vi "GeoData.vi"() -> ()   [LabVIEW 2017] (continued)
H1\n88058\t35013\tSan miguel\tNM\tDona Ana County\tH1\n88001\t35013\tLas cruces\tNM\tDona Ana County\tH1\n88011\t35013\tLas cruces\tNM\tDona Ana County\tH1\n88002\t35013\tWhite sands missile range\tNM\tDona Ana County\tH1\n88008\t35013\tSanta teresa\tNM\tDona Ana County\tH1\n88072\t35013\tVado\tNM\tDona Ana County\tH1\n88013\t35013\tLas cruces\tNM\tDona Ana County\tH1\n88046\t35013\tMesilla\tNM\tDona Ana County\tH1\n88052\t35013\tOrgan\tNM\tDona Ana County\tH1\n88033\t35013\tFairacres\tNM\tDona Ana County\tH1\n87936\t35013\tGarfield\tNM\tDona Ana County\tH1\n88032\t35013\tDona ana\tNM\tDona Ana County\tH1\n88048\t35013\tMesquite\tNM\tDona Ana County\tH1\n88003\t35013\tLas cruces\tNM\tDona Ana County\tH1\n87941\t35013\tSalem\tNM\tDona Ana County\tH1\n88012\t35013\tLas cruces\tNM\tDona Ana County\tH1\n88024\t35013\tBerino\tNM\tDona Ana County\tH1\n88210\t35015\tArtesia\tNM\tEddy County\tH1\n88253\t35015\tLake arthur\tNM\tEddy County\tH1\n88263\t35015\tMalaga\tNM\tEddy County\tH1\n88221\t35015\tCarlsbad\tNM\tEddy County\tH1\n88255\t35015\tLoco hills\tNM\tEddy County\tH1\n88250\t35015\tHope\tNM\tEddy County\tH1\n88268\t35015\tWhites city\tNM\tEddy County\tH1\n88220\t35015\tCarlsbad\tNM\tEddy County\tH1\n88256\t35015\tLoving\tNM\tEddy County\tH1\n88254\t35015\tLakewood\tNM\tEddy County\tH1\n88043\t35017\tHurley\tNM\tGrant County\tH1\n88023\t35017\tBayard\tNM\tGrant County\tH1\n88028\t35017\tCliff\tNM\tGrant County\tH1\n88026\t35017\tSanta clara\tNM\tGrant County\tH1\n88041\t35017\tHanover\tNM\tGrant County\tH1\n88049\t35017\tMimbres\tNM\tGrant County\tH1\n88062\t35017\tSilver city\tNM\tGrant County\tH1\n88055\t35017\tRedrock\tNM\tGrant County\tH1\n88065\t35017\tTyrone\tNM\tGrant County\tH1\n88061\t35017\tSilver city\tNM\tGrant County\tH1\n88025\t35017\tBuckhorn\tNM\tGrant County\tH1\n88034\t35017\tFaywood\tNM\tGrant County\tH1\n88051\t35017\tMule creek\tNM\tGrant County\tH1\n88036\t35017\tFort bayard\tNM\tGrant County\tH1\n88022\t35017\tArenas valley\tNM\tGrant County\tH1\n87821\t35017\tDatil\tNM\tGrant County\tH1\n88040\t35017\tHachita\tNM\tGrant County\tH1\n88053\t35017\tPinos altos\tNM\tGrant County\tH1\n88038\t35017\tGila\tNM\tGrant County\tH1\n88431\t35019\tNewkirk\tNM\tGuadalupe County\tH1\n88353\t35019\tVaughn\tNM\tGuadalupe County\tH1\n88417\t35019\tCuervo\tNM\tGuadalupe County\tH1\n87724\t35019\tLa loma\tNM\tGuadalupe County\tH1\n88435\t35019\tSanta rosa\tNM\tGuadalupe County\tH1\n87711\t35019\tAnton chico\tNM\tGuadalupe County\tH1\n87746\t35021\tSolano\tNM\tHarding County\tH1\n87733\t35021\tMosquero\tNM\tHarding County\tH1\n88415\t35021\tClayton\tNM\tHarding County\tH1\n88410\t35021\tAmistad\tNM\tHarding County\tH1\n88430\t35021\tNara visa\tNM\tHarding County\tH1\n88426\t35021\tLogan\tNM\tHarding County\tH1\n87730\t35021\tMills\tNM\tHarding County\tH1\n87743\t35021\tRoy\tNM\tHarding County\tH1\n88056\t35023\tRodeo\tNM\tHidalgo County\tH1\n88020\t35023\tAnimas\tNM\tHidalgo County\tH1\n88045\t35023\tLordsburg\tNM\tHidalgo County\tH1\n88267\t35025\tTatum\tNM\tLea County\tH1\n88260\t35025\tLovington\tNM\tLea County\tH1\n88213\t35025\tCaprock\tNM\tLea County\tH1\n88114\t35025\tCrossroads\tNM\tLea County\tH1\n88265\t35025\tMonument\tNM\tLea County\tH1\n88264\t35025\tMaljamar\tNM\tLea County\tH1\n88252\t35025\tJal\tNM\tLea County\tH1\n88241\t35025\tHobbs\tNM\tLea County\tH1\n88231\t35025\tEunice\tNM\tLea County\tH1\n88242\t35025\tHobbs\tNM\tLea County\tH1\n88240\t35025\tHobbs\tNM\tLea County\tH1\n88262\t35025\tMcdonald\tNM\tLea County\tH1\n88348\t35027\tSan patricio\tNM\tLincoln County\tH1\n88336\t35027\tHondo\tNM\tLincoln County\tH1\n88323\t35027\tFort stanton\tNM\tLincoln County\tH1\n88324\t35027\tGlencoe\tNM\tLincoln County\tH1\n88318\t35027\tCorona\tNM\tLincoln County\tH1\n88345\t35027\tRuidoso\tNM\tLincoln County\tH1\n88316\t35027\tCapitan\tNM\tLincoln County\tH1\n88355\t35027\tRuidoso\tNM\tLincoln County\tH1\n88301\t35027\tCarrizozo\tNM\tLincoln County\tH1\n88341\t35027\tNogal\tNM\tLincoln County\tH1\n88338\t35027\tLincoln\tNM\tLincoln County\tH1\n88346\t35027\tRuidoso downs\tNM\tLincoln County\tH1\n88312\t35027\tAlto\tNM\tLincoln County\tH1\n88351\t35027\tTinnie\tNM\tLincoln County\tH1\n88343\t35027\tPicacho\tNM\tLincoln County\tH1\n87547\t35028\tWhite rock\tNM\tLos Alamos County\tH1\n87544\t35028\tLos alamos\tNM\tLos Alamos County\tH1\n88030\t35029\tDeming\tNM\tLuna County\tH1\n88029\t35029\tColumbus\tNM\tLuna County\tH1\n88031\t35029\tDeming\tNM\tLuna County\tH1\n87020\t35031\tGrants\tNM\tMcKinley County\tH1\n87316\t35031\tFort wingate\tNM\tMcKinley County\tH1\n87328\t35031\tNavajo\tNM\tMcKinley County\tH1\n87313\t35031\tCrownpoint\tNM\tMcKinley County\tH1\n87319\t35031\tMentmore\tNM\tMcKinley County\tH1\n87323\t35031\tThoreau\tNM\tMcKinley County\tH1\n87321\t35031\tRamah\tNM\tMcKinley County\tH1\n87312\t35031\tContinental divide\tNM\tMcKinley County\tH1\n87311\t35031\tChurch rock\tNM\tMcKinley County\tH1\n87365\t35031\tSmith lake\tNM\tMcKinley County\tH1\n87322\t35031\tRehoboth\tNM\tMcKinley County\tH1\n87347\t35031\tJamestown\tNM\tMcKinley County\tH1\n87327\t35031\tZuni\tNM\tMcKinley County\tH1\n87045\t35031\tPrewitt\tNM\tMcKinley County\tH1\n87326\t35031\tVanderwagen\tNM\tMcKinley County\tH1\n87301\t35031\tGallup\tNM\tMcKinley County\tH1\n87305\t35031\tGallup\tNM\tMcKinley County\tH1\n87310\t35031\tBrimhall\tNM\tMcKinley County\tH1\n87302\t35031\tGallup\tNM\tMcKinley County\tH1\n87317\t35031\tGamerco\tNM\tMcKinley County\tH1\n87325\t35031\tTohatchi\tNM\tMcKinley County\tH1\n87320\t35031\tMexican springs\tNM\tMcKinley County\tH1\n87713\t35033\tChacon\tNM\tMora County\tH1\n87723\t35033\tHolman\tNM\tMora County\tH1\n87736\t35033\tRainsville\tNM\tMora County\tH1\n87715\t35033\tCleveland\tNM\tMora County\tH1\n87734\t35033\tOcate\tNM\tMora County\tH1\n87753\t35033\tWatrous\tNM\tMora County\tH1\n87752\t35033\tWagon mound\tNM\tMora County\tH1\n87732\t35033\tMora\tNM\tMora County\tH1\n87722\t35033\tGuadalupita\tNM\tMora County\tH1\n87735\t35033\tOjo feliz\tNM\tMora County\tH1\n87712\t35033\tBuena vista\tNM\tMora County\tH1\n87750\t35033\tValmora\tNM\tMora County\tH1\n88081\t35035\tChaparral\tNM\tOtero County\tH1\n88314\t35035\tBent\tNM\tOtero County\tH1\n88347\t35035\tSacramento\tNM\tOtero County\tH1\n88317\t35035\tCloudcroft\tNM\tOtero County\tH1\n88325\t35035\tHigh rolls mountain park\tNM\tOtero County\tH1\n88352\t35035\tTularosa\tNM\tOtero County\tH1\n88021\t35035\tAnthony\tNM\tOtero County\tH1\n88344\t35035\tPinon\tNM\tOtero County\tH1\n88340\t35035\tMescalero\tNM\tOtero County\tH1\n88350\t35035\tTimberon\tNM\tOtero County\tH1\n88310\t35035\tAlamogordo\tNM\tOtero County\tH1\n88311\t35035\tAlamogordo\tNM\tOtero County\tH1\n88349\t35035\tSunspot\tNM\tOtero County\tH1\n88342\t35035\tOrogrande\tNM\tOtero County\tH1\n88330\t35035\tHolloman air force base\tNM\tOtero County\tH1\n88337\t35035\tLa luz\tNM\tOtero County\tH1\n88339\t35035\tMayhill\tNM\tOtero County\tH1\n88354\t35035\tWeed\tNM\tOtero County\tH1\n88124\t35037\tMelrose\tNM\tQuay County\tH1\n88433\t35037\tQuay\tNM\tQuay County\tH1\n88120\t35037\tGrady\tNM\tQuay County\tH1\n88434\t35037\tSan jon\tNM\tQuay County\tH1\n88427\t35037\tMcalister\tNM\tQuay County\tH1\n88430\t35037\tNara visa\tNM\tQuay County\tH1\n88426\t35037\tLogan\tNM\tQuay County\tH1\n88411\t35037\tBard\tNM\tQuay County\tH1\n88121\t35037\tHouse\tNM\tQuay County\tH1\n88401\t35037\tTucumcari\tNM\tQuay County\tH1\n88112\t35037\tBroadview\tNM\tQuay County\tH1\n87528\t35039\tDulce\tNM\tRio Arriba County\tH1\n87531\t35039\tEmbudo\tNM\tRio Arriba County\tH1\n87029\t35039\tLindrith\tNM\tRio Arriba County\tH1\n87575\t35039\tTierra amarilla\tNM\tRio Arriba County\tH1\n87523\t35039\tCordova\tNM\tRio Arriba County\tH1\n87522\t35039\tChimayo\tNM\tRio Arriba County\tH1\n87510\t35039\tAbiquiu\tNM\tRio Arriba County\tH1\n87012\t35039\tCoyote\tNM\tRio Arriba County\tH1\n87532\t35039\tEspanola\tNM\tRio Arriba County\tH1\n87566\t35039\tOhkay owingeh\tNM\tRio Arriba County\tH1\n87530\t35039\tEl rito\tNM\tRio Arriba County\tH1\n87548\t35039\tMedanales\tNM\tRio Arriba County\tH1\n87554\t35039\tPetaca\tNM\tRio Arriba County\tH1\n87017\t35039\tGallina\tNM\tRio Arriba County\tH1\n87539\t35039\tLa madera\tNM\tRio Arriba County\tH1\n87520\t35039\tChama\tNM\tRio Arriba County\tH1\n87537\t35039\tHernandez\tNM\tRio Arriba County\tH1\n87551\t35039\tLos ojos\tNM\tRio Arriba County\tH1\n87582\t35039\tVelarde\tNM\tRio Arriba County\tH1\n87064\t35039\tYoungsville\tNM\tRio Arriba County\tH1\n87527\t35039\tDixon\tNM\tRio Arriba County\tH1\n87515\t35039\tCanjilon\tNM\tRio Arriba County\tH1\n87506\t35039\tSanta fe\tNM\tRio Arriba County\tH1\n87046\t35039\tRegina\tNM\tRio Arriba County\tH1\n87518\t35039\tCebolla\tNM\tRio Arriba County\tH1\n87412\t35039\tBlanco\tNM\tRio Arriba County\tH1\n87581\t35039\tVallecitos\tNM\tRio Arriba County\tH1\n87578\t35039\tTruchas\tNM\tRio Arriba County\tH1\n87516\t35039\tCanones\tNM\tRio Arriba County\tH1\n87511\t35039\tAlcalde\tNM\tRio Arriba County\tH1\n88115\t35041\tDora\tNM\tRoosevelt County\tH1\n88124\t35041\tMelrose\tNM\tRoosevelt County\tH1\n88134\t35041\tTaiban\tNM\tRoosevelt County\tH1\n88126\t35041\tPep\tNM\tRoosevelt County\tH1\n88123\t35041\tLingo\tNM\tRoosevelt County\tH1\n88101\t35041\tClovis\tNM\tRoosevelt County\tH1\n88130\t35041\tPortales\tNM\tRoosevelt County\tH1\n88114\t35041\tCrossroads\tNM\tRoosevelt County\tH1\n88113\t35041\tCausey\tNM\tRoosevelt County\tH1\n88125\t35041\tMilnesand\tNM\tRoosevelt County\tH1\n88116\t35041\tElida\tNM\tRoosevelt County\tH1\n88132\t35041\tRogers\tNM\tRoosevelt County\tH1\n88122\t35041\tKenna\tNM\tRoosevelt County\tH1\n88135\t35041\tTexico\tNM\tRoosevelt County\tH1\n88118\t35041\tFloyd\tNM\tRoosevelt County\tH1\n87041\t35043\tPena blanca\tNM\tSandoval County\tH1\n87072\t35043\tCochiti pueblo\tNM\tSandoval County\tH1\n87047\t35043\tSandia park\tNM\tSandoval County\tH1\n87048\t35043\tCorrales\tNM\tSandoval County\tH1\n87544\t35043\tLos alamos\tNM\tSandoval County\tH1\n87025\t35043\tJemez springs\tNM\tSandoval County\tH1\n87053\t35043\tSan ysidro\tNM\tSandoval County\tH1\n87122\t35043\tAlbuquerque\tNM\tSandoval County\tH1\n87174\t35043\tRio rancho\tNM\tSandoval County\tH1\n87124\t35043\tRio rancho\tNM\tSandoval County\tH1\n87027\t35043\tLa jara\tNM\tSandoval County\tH1\n87044\t35043\tPonderosa\tNM\tSandoval County\tH1\n87004\t35043\tBernalillo\tNM\tSandoval County\tH1\n87024\t35043\tJemez pueblo\tNM\tSandoval County\tH1\n87001\t35043\tAlgodones\tNM\tSandoval County\tH1\n87083\t35043\tCochiti lake\tNM\tSandoval County\tH1\n87043\t35043\tPlacitas\tNM\tSandoval County\tH1\n87052\t35043\tSanto domingo pueblo\tNM\tSandoval County\tH1\n87018\t35043\tCounselor\tNM\tSandoval County\tH1\n87046\t35043\tRegina\tNM\tSandoval County\tH1\n87144\t35043\tRio rancho\tNM\tSandoval County\tH1\n87013\t35043\tCuba\tNM\tSandoval County\tH1\n87402\t35045\tFarmington\tNM\tSan Juan County\tH1\n87499\t35045\tFarmington\tNM\tSan Juan County\tH1\n87418\t35045\tLa plata\tNM\tSan Juan County\tH1\n87455\t35045\tNewcomb\tNM\tSan Juan County\tH1\n87421\t35045\tWaterflow\tNM\tSan Juan County\tH1\n87419\t35045\tNavajo dam\tNM\tSan Juan County\tH1\n87461\t35045\tSanostee\tNM\tSan Juan County\tH1\n87413\t35045\tBloomfield\tNM\tSan Juan County\tH1\n87420\t35045\tShiprock\tNM\tSan Juan County\tH1\n87416\t35045\tFruitland\tNM\tSan Juan County\tH1\n87417\t35045\tKirtland\tNM\tSan Juan County\tH1\n87364\t35045\tSheep springs\tNM\tSan Juan County\tH1\n87037\t35045\tNageezi\tNM\tSan Juan County\tH1\n87412\t35045\tBlanco\tNM\tSan Juan County\tH1\n87401\t35045\tFarmington\tNM\tSan Juan County\tH1\n87410\t35045\tAztec\tNM\tSan Juan County\tH1\n87415\t35045\tFlora vista\tNM\tSan Juan County\tH1\n87565\t35047\tSan jose\tNM\tSan Miguel County\tH1\n87746\t35047\tSolano\tNM\tSan Miguel County\tH1\n87583\t35047\tVillanueva\tNM\tSan Miguel County\tH1\n88421\t35047\tGarita\tNM\tSan Miguel County\tH1\n87569\t35047\tSerafina\tNM\tSan Miguel County\tH1\n87538\t35047\tIlfeld\tNM\tSan Miguel County\tH1\n87560\t35047\tRibera\tNM\tSan Miguel County\tH1\n87573\t35047\tTererro\tNM\tSan Miguel County\tH1\n87701\t35047\tLas vegas\tNM\tSan Miguel County\tH1\n87552\t35047\tPecos\tNM\tSan Miguel County\tH1\n88439\t35047\tTrementina\tNM\tSan Miguel County\tH1\n87562\t35047\tRowe\tNM\tSan Miguel County\tH1\n87731\t35047\tMontezuma\tNM\tSan Miguel County\tH1\n88416\t35047\tConchas dam\tNM\tSan Miguel County\tH1\n87711\t35047\tAnton chico\tNM\tSan Miguel County\tH1\n87535\t35047\tGlorieta\tNM\tSan Miguel County\tH1\n87745\t35047\tSapello\tNM\tSan Miguel County\tH1\n87742\t35047\tRociada\tNM\tSan Miguel County\tH1\n87035\t35049\tMoriarty\tNM\tSanta Fe County\tH1\n87502\t35049\tSanta fe\tNM\tSanta Fe County\tH1\n87015\t35049\tEdgewood\tNM\tSanta Fe County\tH1\n87047\t35049\tSandia park\tNM\tSanta Fe County\tH1\n87504\t35049\tSanta fe\tNM\tSanta Fe County\tH1\n87522\t35049\tChimayo\tNM\tSanta Fe County\tH1\n87567\t35049\tSanta cruz\tNM\tSanta Fe County\tH1\n87505\t35049\tSanta fe\tNM\tSanta Fe County\tH1\n87532\t35049\tEspanola\tNM\tSanta Fe County\tH1\n87592\t35049\tSanta fe\tNM\tSanta Fe County\tH1\n87501\t35049\tSanta fe\tNM\tSanta Fe County\tH1\n87540\t35049\tLamy\tNM\tSanta Fe County\tH1\n87010\t35049\tCerrillos\tNM\tSanta Fe County\tH1\n87508\t35049\tSanta fe\tNM\tSanta Fe County\tH1\n87552\t35049\tPecos\tNM\tSanta Fe County\tH1\n87506\t35049\tSanta fe\tNM\tSanta Fe County\tH1\n87507\t35049\tSanta fe\tNM\tSanta Fe County\tH1\n87594\t35049\tSanta fe\tNM\tSanta Fe County\tH1\n87056\t35049\tStanley\tNM\tSanta Fe County\tH1\n87574\t35049\tTesuque\tNM\tSanta Fe County\tH1\n87535\t35049\tGlorieta\tNM\tSanta Fe County\tH1\n87901\t35051\tTruth or consequences\tNM\tSierra County\tH1\n87942\t35051\tWilliamsburg\tNM\tSierra County\tH1\n87654\t35051\tSpaceport city\tNM\tSierra County\tH1\n87930\t35051\tArrey\tNM\tSierra County\tH1\n87933\t35051\tDerry\tNM\tSierra County\tH1\n87943\t35051\tWinston\tNM\tSierra County\tH1\n87931\t35051\tCaballo\tNM\tSierra County\tH1\n87935\t35051\tElephant butte\tNM\tSierra County\tH1\n88042\t35051\tHillsboro\tNM\tSierra County\tH1\n87939\t35051\tMonticello\tNM\tSierra County\tH1\n87823\t35053\tLemitar\tNM\tSocorro County\tH1\n87825\t35053\tMagdalena\tNM\tSocorro County\tH1\n87801\t35053\tSocorro\tNM\tSocorro County\tH1\n87028\t35053\tLa joya\tNM\tSocorro County\tH1\n87011\t35053\tClaunch\tNM\tSocorro County\tH1\n87062\t35053\tVeguita\tNM\tSocorro County\tH1\n87006\t35053\tBosque\tNM\tSocorro County\tH1\n87828\t35053\tPolvadera\tNM\tSocorro County\tH1\n87831\t35053\tSan acacia\tNM\tSocorro County\tH1\n87832\t35053\tSan antonio\tNM\tSocorro County\tH1\n87514\t35055\tArroyo seco\tNM\tTaos County\tH1\n87524\t35055\tCostilla\tNM\tTaos County\tH1\n87577\t35055\tTres piedras\tNM\tTaos County\tH1\n87576\t35055\tTrampas\tNM\tTaos County\tH1\n87579\t35055\tVadito\tNM\tTaos County\tH1\n87580\t35055\tValdez\tNM\tTaos County\tH1\n87525\t35055\tTaos ski valley\tNM\tTaos County\tH1\n87571\t35055\tTaos\tNM\tTaos County\tH1\n87519\t35055\tCerro\tNM\tTaos County\tH1\n87543\t35055\tLlano\tNM\tTaos County\tH1\n87512\t35055\tAmalia\tNM\tTaos County\tH1\n87553\t35055\tPenasco\tNM\tTaos County\tH1\n87558\t35055\tRed river\tNM\tTaos County\tH1\n87549\t35055\tOjo caliente\tNM\tTaos County\tH1\n87557\t35055\tRanchos de taos\tNM\tTaos County\tH1\n87529\t35055\tEl prado\tNM\tTaos County\tH1\n87521\t35055\tChamisal\tNM\tTaos County\tH1\n87513\t35055\tArroyo hondo\tNM\tTaos County\tH1\n87517\t35055\tCarson\tNM\tTaos County\tH1\n87564\t35055\tSan cristobal\tNM\tTaos County\tH1\n87556\t35055\tQuesta\tNM\tTaos County\tH1\n87035\t35057\tMoriarty\tNM\tTorrance County\tH1\n87015\t35057\tEdgewood\tNM\tTorrance County\tH1\n87061\t35057\tTorreon\tNM\tTorrance County\tH1\n87070\t35057\tClines corners\tNM\tTorrance County\tH1\n88321\t35057\tEncino\tNM\tTorrance County\tH1\n87009\t35057\tCedarvale\tNM\tTorrance County\tH1\n87016\t35057\tEstancia\tNM\tTorrance County\tH1\n87036\t35057\tMountainair\tNM\tTorrance County\tH1\n87063\t35057\tWillard\tNM\tTorrance County\tH1\n87032\t35057\tMcintosh\tNM\tTorrance County\tH1\n88414\t35059\tCapulin\tNM\tUnion County\tH1\n88415\t35059\tClayton\tNM\tUnion County\tH1\n88410\t35059\tAmistad\tNM\tUnion County\tH1\n88422\t35059\tGladstone\tNM\tUnion County\tH1\n88419\t35059\tFolsom\tNM\tUnion County\tH1\n88418\t35059\tDes moines\tNM\tUnion County\tH1\n88430\t35059\tNara visa\tNM\tUnion County\tH1\n88436\t35059\tSedan\tNM\tUnion County\tH1\n88424\t35059\tGrenville\tNM\tUnion County\tH1\n87031\t35061\tLos lunas\tNM\tValencia County\tH1\n87068\t35061\tBosque farms\tNM\tValencia County\tH1\n87060\t35061\tTome\tNM\tValencia County\tH1\n87042\t35061\tPeralta\tNM\tValencia County\tH1\n87062\t35061\tVeguita\tNM\tValencia County\tH1\n87006\t35061\tBosque\tNM\tValencia County\tH1\n87002\t35061\tBelen\tNM\tValencia County\tH1\n87026\t35061\tLaguna\tNM\tValencia County\tH1\n87023\t35061\tJarales\tNM\tValencia County\tH1\n12087\t36001\tHannacroix\tNY\tAlbany County\tH1\n12189\t36001\tWatervliet\tNY\tAlbany County\tH1\n12204\t36001\tAlbany\tNY\tAlbany County\tH1\n12207\t36001\tAlbany\tNY\tAlbany County\tH1\n12226\t36001\tAlbany\tNY\tAlbany County\tH1\n12234\t36001\tAlbany\tNY\tAlbany County\tH1\n12232\t36001\tAlbany\tNY\tAlbany County\tH1\n12055\t36001\tDormansville\tNY\tAlbany County\tH1\n12469\t36001\tPreston hollow\tNY\tAlbany County\tH1\n12047\t36001\tCohoes\tNY\tAlbany County\tH1\n12157\t36001\tSchoharie\tNY\tAlbany County\tH1\n12183\t36001\tTroy\tNY\tAlbany County\tH1\n12007\t36001\tAlcove\tNY\tAlbany County\tH1\n12041\t36001\tClarksville\tNY\tAlbany County\tH1\n12255\t36001\tAlbany\tNY\tAlbany County\tH1\n12460\t36001\tOak hill\tNY\tAlbany County\tH1\n12023\t36001\tBerne\tNY\tAlbany County\tH1\n12053\t36001\tDelanson\tNY\tAlbany County\tH1\n12161\t36001\tSouth bethlehem\tNY\tAlbany County\tH1\n12122\t36001\tMiddleburgh\tNY\tAlbany County\tH1\n12206\t36001\tAlbany\tNY\tAlbany County\tH1\n12306\t36001\tSchenectady\tNY\tAlbany County\tH1\n12257\t36001\tAlbany\tNY\tAlbany County\tH1\n12107\t36001\tKnox\tNY\tAlbany County\tH1\n12245\t36001\tAlbany\tNY\tAlbany County\tH1\n12083\t36001\tGreenville\tNY\tAlbany County\tH1\n12158\t36001\tSelkirk\tNY\tAlbany County\tH1\n12205\t36001\tAlbany\tNY\tAlbany County\tH1\n12309\t36001\tSchenectady\tNY\tAlbany County\tH1\n12247\t36001\tAlbany\tNY\tAlbany County\tH1\n12223\t36001\tAlbany\tNY\tAlbany County\tH1\n12222\t36001\tAlbany\tNY\tAlbany County\tH1\n12260\t36001\tAlbany\tNY\tAlbany County\tH1\n12235\t36001\tAlbany\tNY\tAlbany County\tH1\n12249\t36001\tAlbany\tNY\tAlbany County\tH1\n12110\t36001\tLatham\tNY\tAlbany County\tH1\n12159\t36001\tSlingerlands\tNY\tAlbany County\tH1\n12202\t36001\tAlbany\tNY\tAlbany County\tH1\n12193\t36001\tWesterlo\tNY\tAlbany County\tH1\n12067\t36001\tFeura bush\tNY\tAlbany County\tH1\n12077\t36001\tGlenmont\tNY\tAlbany County\tH1\n12084\t36001\tGuilderland\tNY\tAlbany County\tH1\n12059\t36001\tEast berne\tNY\tAlbany County\tH1\n12147\t36001\tRensselaerville\tNY\tAlbany County\tH1\n12143\t36001\tRavena\tNY\tAlbany County\tH1\n12186\t36001\tVoorheesville\tNY\tAlbany County\tH1\n12209\t36001\tAlbany\tNY\tAlbany County\tH1\n12303\t36001\tSchenectady\tNY\tAlbany County\tH1\n12304\t36001\tSchenectady\tNY\tAlbany County\tH1\n12045\t36001\tCoeymans\tNY\tAlbany County\tH1\n12120\t36001\tMedusa\tNY\tAlbany County\tH1\n12085\t36001\tGuilderland center\tNY\tAlbany County\tH1\n12240\t36001\tAlbany\tNY\tAlbany County\tH1\n12248\t36001\tAlbany\tNY\tAlbany County\tH1\n12128\t36001\tNewtonville\tNY\tAlbany County\tH1\n12224\t36001\tAlbany\tNY\tAlbany County\tH1\n12009\t36001\tAltamont\tNY\tAlbany County\tH1\n12208\t36001\tAlbany\tNY\tAlbany County\tH1\n12212\t36001\tAlbany\tNY\tAlbany County\tH1\n12201\t36001\tAlbany\tNY\tAlbany County\tH1\n12236\t36001\tAlbany\tNY\tAlbany County\tH1\n12054\t36001\tDelmar\tNY\tAlbany County\tH1\n12065\t36001\tClifton park\tNY\tAlbany County\tH1\n12203\t36001\tAlbany\tNY\tAlbany County\tH1\n12211\t36001\tAlbany\tNY\tAlbany County\tH1\n12210\t36001\tAlbany\tNY\tAlbany County\tH1\n12046\t36001\tCoeymans hollow\tNY\tAlbany County\tH1\n12220\t36001\tAlbany\tNY\tAlbany County\tH1\n12246\t36001\tAlbany\tNY\tAlbany County\tH1\n12237\t36001\tAlbany\tNY\tAlbany County\tH1\n12288\t36001\tAlbany\tNY\tAlbany County\tH1\n12227\t36001\tAlbany\tNY\tAlbany County\tH1\n14717\t36003\tCaneadea\tNY\tAllegany County\tH1\n14802\t36003\tAlfred\tNY\tAllegany County\tH1\n14060\t36003\tFarmersville station\tNY\tAllegany County\tH1\n14721\t36003\tCeres\tNY\tAllegany County\tH1\n14745\t36003\tHume\tNY\tAllegany County\tH1\n14065\t36003\tFreedom\tNY\tAllegany County\tH1\n14822\t36003\tCanaseraga\tNY\tAllegany County\tH1\n14836\t36003\tDalton\tNY\tAllegany County\tH1\n14843\t36003\tHornell\tNY\tAllegany County\tH1\n14897\t36003\tWhitesville\tNY\tAllegany County\tH1\n14029\t36003\tCenterville\tNY\tAllegany County\tH1\n14774\t36003\tRichburg\tNY\tAllegany County\tH1\n14754\t36003\tLittle genesee\tNY\tAllegany County\tH1\n14709\t36003\tAngelica\tNY\tAllegany County\tH1\n14884\t36003\tSwain\tNY\tAllegany County\tH1\n14714\t36003\tBlack creek\tNY\tAllegany County\tH1\n14895\t36003\tWellsville\tNY\tAllegany County\tH1\n14806\t36003\tAndover\tNY\tAllegany County\tH1\n14786\t36003\tWest clarksville\tNY\tAllegany County\tH1\n14437\t36003\tDansville\tNY\tAllegany County\tH1\n14803\t36003\tAlfred station\tNY\tAllegany County\tH1\n14715\t36003\tBolivar\tNY\tAllegany County\tH1\n14708\t36003\tAlma\tNY\tAllegany County\tH1\n14024\t36003\tBliss\tNY\tAllegany County\tH1\n14727\t36003\tCuba\tNY\tAllegany County\tH1\n14770\t36003\tPortville\tNY\tAllegany County\tH1\n14807\t36003\tArkport\tNY\tAllegany County\tH1\n14739\t36003\tFriendship\tNY\tAllegany County\tH1\n14846\t36003\tHunt\tNY\tAllegany County\tH1\n14744\t36003\tHoughton\tNY\tAllegany County\tH1\n14707\t36003\tAllentown\tNY\tAllegany County\tH1\n14737\t36003\tFranklinville\tNY\tAllegany County\tH1\n14813\t36003\tBelmont\tNY\tAllegany County\tH1\n14735\t36003\tFillmore\tNY\tAllegany County\tH1\n14880\t36003\tScio\tNY\tAllegany County\tH1\n14777\t36003\tRushford\tNY\tAllegany County\tH1\n14804\t36003\tAlmond\tNY\tAllegany County\tH1\n14711\t36003\tBelfast\tNY\tAllegany County\tH1\n14536\t36003\tPortageville\tNY\tAllegany County\tH1\n10459\t36005\tBronx\tNY\tBronx County\tH6\n10457\t36005\tBronx\tNY\tBronx County\tH6\n10455\t36005\tBronx\tNY\tBronx County\tH6\n10465\t36005\tBronx\tNY\tBronx County\tH6\n10468\t36005\tBronx\tNY\tBronx County\tH6\n10466\t36005\tBronx\tNY\tBronx County\tH6\n10473\t36005\tBronx\tNY\tBronx County\tH6\n10550\t36005\tMount vernon\tNY\tBronx County\tH6\n10458\t36005\tBronx\tNY\tBronx County\tH6\n10463\t36005\tBronx\tNY\tBronx County\tH6\n10464\t36005\tBronx\tNY\tBronx County\tH6\n10469\t36005\tBronx\tNY\tBronx County\tH6\n10453\t36005\tBronx\tNY\tBronx County\tH6\n10460\t36005\tBronx\tNY\tBronx County\tH6\n10461\t36005\tBronx\tNY\tBronx County\tH6\n10462\t36005\tBronx\tNY\tBronx County\tH6\n10471\t36005\tBronx\tNY\tBronx County\tH6\n10454\t36005\tBronx\tNY\tBronx County\tH6\n10456\t36005\tBronx\tNY\tBronx County\tH6\n10467\t36005\tBronx\tNY\tBronx County\tH6\n10470\t36005\tBronx\tNY\tBronx County\tH6\n10475\t36005\tBronx\tNY\tBronx County\tH6\n10472\t36005\tBronx\tNY\tBronx County\tH6\n10474\t36005\tBronx\tNY\tBronx County\tH6\n10705\t36005\tYonkers\tNY\tBronx County\tH6\n10452\t36005\tBronx\tNY\tBronx County\tH6\n10451\t36005\tBronx\tNY\tBronx County\tH6\n10803\t36005\tPelham\tNY\tBronx County\tH6\n13746\t36007\tChenango forks\tNY\tBroome County\tH1\n13730\t36007\tAfton\tNY\tBroome County\tH1\n13787\t36007\tHarpursville\tNY\tBroome County\tH1\n13850\t36007\tVestal\tNY\tBroome County\tH1\n13901\t36007\tBinghamton\tNY\tBroome County\tH1\n13835\t36007\tRichford\tNY\tBroome County\tH1\n13813\t36007\tNineveh\tNY\tBroome County\tH1\n13732\t36007\tApalachin\tNY\tBroome County\tH1\n13778\t36007\tGreene\tNY\tBroome County\tH1\n13761\t36007\tEndicott\tNY\tBroome County\tH1\n13797\t36007\tLisle\tNY\tBroome County\tH1\n13803\t36007\tMarathon\tNY\tBroome County\tH1\n13777\t36007\tGlen aubrey\tNY\tBroome County\tH1\n13737\t36007\tBible school park\tNY\tBroome County\tH1\n13790\t36007\tJohnson city\tNY\tBroome County\tH1\n13902\t36007\tBinghamton\tNY\tBroome County\tH1\n13762\t36007\tEndwell\tNY\tBroome County\tH1\n13754\t36007\tDeposit\tNY\tBroome County\tH1\n13736\t36007\tBerkshire\tNY\tBroome County\tH1\n13811\t36007\tNewark valley\tNY\tBroome County\tH1\n13745\t36007\tChenango bridge\tNY\tBroome County\tH1\n13794\t36007\tKillawog\tNY\tBroome County\tH1\n13851\t36007\tVestal\tNY\tBroome County\tH1\n13833\t36007\tPort crane\tNY\tBroome County\tH1\n13904\t36007\tBinghamton\tNY\tBroome County\tH1\n13795\t36007\tKirkwood\tNY\tBroome County\tH1\n13748\t36007\tConklin\tNY\tBroome County\tH1\n13760\t36007\tEndicott\tNY\tBroome County\tH1\n13802\t36007\tMaine\tNY\tBroome County\tH1\n13862\t36007\tWhitney point\tNY\tBroome County\tH1\n13826\t36007\tOuaquaga\tNY\tBroome County\tH1\n13783\t36007\tHancock\tNY\tBroome County\tH1\n13744\t36007\tCastle creek\tNY\tBroome County\tH1\n13903\t36007\tBinghamton\tNY\tBroome County\tH1\n13905\t36007\tBinghamton\tNY\tBroome County\tH1\n13865\t36007\tWindsor\tNY\tBroome County\tH1\n13863\t36007\tWillet\tNY\tBroome County\tH1\n13848\t36007\tTunnel\tNY\tBroome County\tH1\n13749\t36007\tCorbettsville\tNY\tBroome County\tH1\n14738\t36009\tFrewsburg\tNY\tCattaraugus County\tH1\n14755\t36009\tLittle valley\tNY\tCattaraugus County\tH1\n14134\t36009\tSardinia\tNY\tCattaraugus County\tH1\n14030\t36009\tChaffee\tNY\tCattaraugus County\tH1\n14060\t36009\tFarmersville station\tNY\tCattaraugus County\tH1\n14041\t36009\tDayton\tNY\tCattaraugus County\tH1\n14751\t36009\tLeon\tNY\tCattaraugus County\tH1\n14065\t36009\tFreedom\tNY\tCattaraugus County\tH1\n14729\t36009\tEast otto\tNY\tCattaraugus County\tH1\n14753\t36009\tLimestone\tNY\tCattaraugus County\tH1\n14766\t36009\tOtto\tNY\tCattaraugus County\tH1\n14101\t36009\tMachias\tNY\tCattaraugus County\tH1\n14747\t36009\tKennedy\tNY\tCattaraugus County\tH1\n14779\t36009\tSalamanca\tNY\tCattaraugus County\tH1\n14129\t36009\tPerrysburg\tNY\tCattaraugus County\tH1\n14778\t36009\tSaint bonaventure\tNY\tCattaraugus County\tH1\n14042\t36009\tDelevan\tNY\tCattaraugus County\tH1\n14719\t36009\tCattaraugus\tNY\tCattaraugus County\tH1\n14760\t36009\tOlean\tNY\tCattaraugus County\tH1\n14081\t36009\tIrving\tNY\tCattaraugus County\tH1\n14171\t36009\tWest valley\tNY\tCattaraugus County\tH1\n14706\t36009\tAllegany\tNY\tCattaraugus County\tH1\n14070\t36009\tGowanda\tNY\tCattaraugus County\tH1\n14062\t36009\tForestville\tNY\tCattaraugus County\tH1\n14138\t36009\tSouth dayton\tNY\tCattaraugus County\tH1\n14748\t36009\tKill buck\tNY\tCattaraugus County\tH1\n14783\t36009\tSteamburg\tNY\tCattaraugus County\tH1\n14730\t36009\tEast randolph\tNY\tCattaraugus County\tH1\n14727\t36009\tCuba\tNY\tCattaraugus County\tH1\n14770\t36009\tPortville\tNY\tCattaraugus County\tH1\n14788\t36009\tWestons mills\tNY\tCattaraugus County\tH1\n14009\t36009\tArcade\tNY\tCattaraugus County\tH1\n14737\t36009\tFranklinville\tNY\tCattaraugus County\tH1\n14726\t36009\tConewango valley\tNY\tCattaraugus County\tH1\n14743\t36009\tHinsdale\tNY\tCattaraugus County\tH1\n14741\t36009\tGreat valley\tNY\tCattaraugus County\tH1\n14173\t36009\tYorkshire\tNY\tCattaraugus County\tH1\n14141\t36009\tSpringville\tNY\tCattaraugus County\tH1\n14731\t36009\tEllicottville\tNY\tCattaraugus County\tH1\n14772\t36009\tRandolph\tNY\tCattaraugus County\tH1\n14168\t36009\tVersailles\tNY\tCattaraugus County\tH1\n13074\t36011\tHannibal\tNY\tCayuga County\tH1\n13092\t36011\tLocke\tNY\tCayuga County\tH1\n13111\t36011\tMartville\tNY\tCayuga County\tH1\n13143\t36011\tRed creek\tNY\tCayuga County\tH1\n13166\t36011\tWeedsport\tNY\tCayuga County\tH1\n13024\t36011\tAuburn\tNY\tCayuga County\tH1\n13034\t36011\tCayuga\tNY\tCayuga County\tH1\n13117\t36011\tMontezuma\tNY\tCayuga County\tH1\n13022\t36011\tAuburn\tNY\tCayuga County\tH1\n13027\t36011\tBaldwinsville\tNY\tCayuga County\tH1\n13152\t36011\tSkaneateles\tNY\tCayuga County\tH1\n13160\t36011\tUnion springs\tNY\tCayuga County\tH1\n13071\t36011\tGenoa\tNY\tCayuga County\tH1\n13033\t36011\tCato\tNY\tCayuga County\tH1\n13080\t36011\tJordan\tNY\tCayuga County\tH1\n13147\t36011\tScipio center\tNY\tCayuga County\tH1\n14882\t36011\tLansing\tNY\tCayuga County\tH1\n13026\t36011\tAurora\tNY\tCayuga County\tH1\n13113\t36011\tMeridian\tNY\tCayuga County\tH1\n13045\t36011\tCortland\tNY\tCayuga County\tH1\n13077\t36011\tHomer\tNY\tCayuga County\tH1\n13073\t36011\tGroton\tNY\tCayuga County\tH1\n13146\t36011\tSavannah\tNY\tCayuga County\tH1\n13140\t36011\tPort byron\tNY\tCayuga County\tH1\n13060\t36011\tElbridge\tNY\tCayuga County\tH1\n13126\t36011\tOswego\tNY\tCayuga County\tH1\n13081\t36011\tKing ferry\tNY\tCayuga County\tH1\n13021\t36011\tAuburn\tNY\tCayuga County\tH1\n13156\t36011\tSterling\tNY\tCayuga County\tH1\n13064\t36011\tFair haven\tNY\tCayuga County\tH1\n13139\t36011\tPoplar ridge\tNY\tCayuga County\tH1\n13118\t36011\tMoravia\tNY\tCayuga County\tH1\n14048\t36013\tDunkirk\tNY\tChautauqua County\tH1\n14787\t36013\tWestfield\tNY\tChautauqua County\tH1\n14738\t36013\tFrewsburg\tNY\tChautauqua County\tH1\n14742\t36013\tGreenhurst\tNY\tChautauqua County\tH1\n14758\t36013\tNiobe\tNY\tChautauqua County\tH1\n14701\t36013\tJamestown\tNY\tChautauqua County\tH1\n14750\t36013\tLakewood\tNY\tChautauqua County\tH1\n14767\t36013\tPanama\tNY\tChautauqua County\tH1\n14785\t36013\tStow\tNY\tChautauqua County\tH1\n14723\t36013\tCherry creek\tNY\tChautauqua County\tH1\n14747\t36013\tKennedy\tNY\tChautauqua County\tH1\n14757\t36013\tMayville\tNY\tChautauqua County\tH1\n14775\t36013\tRipley\tNY\tChautauqua County\tH1\n14724\t36013\tClymer\tNY\tChautauqua County\tH1\n14736\t36013\tFindley lake\tNY\tChautauqua County\tH1\n14081\t36013\tIrving\tNY\tChautauqua County\tH1\n14712\t36013\tBemus point\tNY\tChautauqua County\tH1\n14784\t36013\tStockton\tNY\tChautauqua County\tH1\n14728\t36013\tDewittville\tNY\tChautauqua County\tH1\n14063\t36013\tFredonia\tNY\tChautauqua County\tH1\n14782\t36013\tSinclairville\tNY\tChautauqua County\tH1\n14062\t36013\tForestville\tNY\tChautauqua County\tH1\n14138\t36013\tSouth dayton\tNY\tChautauqua County\tH1\n14702\t36013\tJamestown\tNY\tChautauqua County\tH1\n14166\t36013\tVan buren point\tNY\tChautauqua County\tH1\n14752\t36013\tLily dale\tNY\tChautauqua County\tH1\n14710\t36013\tAshville\tNY\tChautauqua County\tH1\n14720\t36013\tCeloron\tNY\tChautauqua County\tH1\n14781\t36013\tSherman\tNY\tChautauqua County\tH1\n14740\t36013\tGerry\tNY\tChautauqua County\tH1\n14135\t36013\tSheridan\tNY\tChautauqua County\tH1\n14136\t36013\tSilver creek\tNY\tChautauqua County\tH1\n14726\t36013\tConewango valley\tNY\tChautauqua County\tH1\n14732\t36013\tEllington\tNY\tChautauqua County\tH1\n14716\t36013\tBrocton\tNY\tChautauqua County\tH1\n14718\t36013\tCassadaga\tNY\tChautauqua County\tH1\n14733\t36013\tFalconer\tNY\tChautauqua County\tH1\n14769\t36013\tPortland\tNY\tChautauqua County\tH1\n14722\t36013\tChautauqua\tNY\tChautauqua County\tH1\n14824\t36015\tCayuta\tNY\tChemung County\tH1\n14905\t36015\tElmira\tNY\tChemung County\tH1\n14904\t36015\tElmira\tNY\tChemung County\tH1\n14812\t36015\tBeaver dams\tNY\tChemung County\tH1\n14889\t36015\tVan etten\tNY\tChemung County\tH1\n14867\t36015\tNewfield\tNY\tChemung County\tH1\n14805\t36015\tAlpine\tNY\tChemung County\tH1\n14825\t36015\tChemung\tNY\tChemung County\tH1\n14901\t36015\tElmira\tNY\tChemung County\tH1\n14845\t36015\tHorseheads\tNY\tChemung County\tH1\n14883\t36015\tSpencer\tNY\tChemung County\tH1\n14903\t36015\tElmira\tNY\tChemung County\tH1\n14859\t36015\tLockwood\tNY\tChemung County\tH1\n14814\t36015\tBig flats\tNY\tChemung County\tH1\n14892\t36015\tWaverly\tNY\tChemung County\tH1\n14861\t36015\tLowman\tNY\tChemung County\tH1\n14816\t36015\tBreesport\tNY\tChemung County\tH1\n14871\t36015\tPine city\tNY\tChemung County\tH1\n14902\t36015\tElmira\tNY\tChemung County\tH1\n14830\t36015\tCorning\tNY\tChemung County\tH1\n14864\t36015\tMillport\tNY\tChemung County\tH1\n14838\t36015\tErin\tNY\tChemung County\tH1\n14872\t36015\tPine valley\tNY\tChemung County\tH1\n14894\t36015\tWellsburg\tNY\tChemung County\tH1\n13746\t36017\tChenango forks\tNY\tChenango County\tH1\n13730\t36017\tAfton\tNY\tChenango County\tH1\n13801\t36017\tMc donough\tNY\tChenango County\tH1\n13780\t36017\tGuilford\tNY\tChenango County\tH1\n13787\t36017\tHarpursville\tNY\tChenango County\tH1\n13830\t36017\tOxford\tNY\tChenango County\tH1\n13813\t36017\tNineveh\tNY\tChenango County\tH1\n13124\t36017\tNorth pitcher\tNY\tChenango County\tH1\n13778\t36017\tGreene\tNY\tChenango County\tH1\n13844\t36017\tSouth plymouth\tNY\tChenango County\tH1\n13841\t36017\tSmithville flats\tNY\tChenango County\tH1\n13460\t36017\tSherburne\tNY\tChenango County\tH1\n13136\t36017\tPitcher\tNY\tChenango County\tH1\n13809\t36017\tMount upton\tNY\tChenango County\tH1\n13814\t36017\tNorth norwich\tNY\tChenango County\tH1\n13758\t36017\tEast pharsalia\tNY\tChenango County\tH1\n13040\t36017\tCincinnatus\tNY\tChenango County\tH1\n13411\t36017\tNew berlin\tNY\tChenango County\tH1\n13485\t36017\tWest edmeston\tNY\tChenango County\tH1\n13733\t36017\tBainbridge\tNY\tChenango County\tH1\n13832\t36017\tPlymouth\tNY\tChenango County\tH1\n13052\t36017\tDe ruyter\tNY\tChenango County\tH1\n13072\t36017\tGeorgetown\tNY\tChenango County\tH1\n13332\t36017\tEarlville\tNY\tChenango County\tH1\n13464\t36017\tSmyrna\tNY\tChenango County\tH1\n13155\t36017\tSouth otselic\tNY\tChenango County\tH1\n13815\t36017\tNorwich\tNY\tChenango County\tH1\n13843\t36017\tSouth new berlin\tNY\tChenango County\tH1\n12981\t36019\tSaranac\tNY\tClinton County\tH1\n12921\t36019\tChazy\tNY\tClinton County\tH1\n12933\t36019\tEllenburg\tNY\tClinton County\tH1\n12903\t36019\tPlattsburgh\tNY\tClinton County\tH1\n12955\t36019\tLyon mountain\tNY\tClinton County\tH1\n12923\t36019\tChurubusco\tNY\tClinton County\tH1\n12997\t36019\tWilmington\tNY\tClinton County\tH1\n12929\t36019\tDannemora\tNY\tClinton County\tH1\n12935\t36019\tEllenburg depot\tNY\tClinton County\tH1\n12985\t36019\tSchuyler falls\tNY\tClinton County\tH1\n12924\t36019\tKeeseville\tNY\tClinton County\tH1\n12919\t36019\tChamplain\tNY\tClinton County\tH1\n12978\t36019\tRedford\tNY\tClinton County\tH1\n12934\t36019\tEllenburg center\tNY\tClinton County\tH1\n12992\t36019\tWest chazy\tNY\tClinton County\tH1\n12979\t36019\tRouses point\tNY\tClinton County\tH1\n12958\t36019\tMooers\tNY\tClinton County\tH1\n12910\t36019\tAltona\tNY\tClinton County\tH1\n12944\t36019\tKeeseville\tNY\tClinton County\tH1\n12918\t36019\tCadyville\tNY\tClinton County\tH1\n12952\t36019\tLyon mountain\tNY\tClinton County\tH1\n12901\t36019\tPlattsburgh\tNY\tClinton County\tH1\n12962\t36019\tMorrisonville\tNY\tClinton County\tH1\n12972\t36019\tPeru\tNY\tClinton County\tH1\n12920\t36019\tChateaugay\tNY\tClinton County\tH1\n12911\t36019\tKeeseville\tNY\tClinton County\tH1\n12913\t36019\tBloomingdale\tNY\tClinton County\tH1\n12959\t36019\tMooers forks\tNY\tClinton County\tH1\n12912\t36019\tAu sable forks\tNY\tClinton County\tH1\n12037\t36021\tChatham\tNY\tColumbia County\tH1\n12075\t36021\tGhent\tNY\tColumbia County\tH1\n12583\t36021\tTivoli\tNY\tColumbia County\tH1\n12195\t36021\tWest lebanon\tNY\tColumbia County\tH1\n12529\t36021\tHillsdale\tNY\tColumbia County\tH1\n12060\t36021\tEast chatham\tNY\tColumbia County\tH1\n12130\t36021\tNiverville\tNY\tColumbia County\tH1\n12184\t36021\tValatie\tNY\tColumbia County\tH1\n12168\t36021\tStephentown\tNY\tColumbia County\tH1\n12115\t36021\tMalden bridge\tNY\tColumbia County\tH1\n12172\t36021\tStottville\tNY\tColumbia County\tH1\n12174\t36021\tStuyvesant falls\tNY\tColumbia County\tH1\n12517\t36021\tCopake falls\tNY\tColumbia County\tH1\n12513\t36021\tClaverack\tNY\tColumbia County\tH1\n12534\t36021\tHudson\tNY\tColumbia County\tH1\n12503\t36021\tAncramdale\tNY\tColumbia County\tH1\n12571\t36021\tRed hook\tNY\tColumbia County\tH1\n12029\t36021\tCanaan\tNY\tColumbia County\tH1\n12123\t36021\tNassau\tNY\tColumbia County\tH1\n12502\t36021\tAncram\tNY\tColumbia County\tH1\n12521\t36021\tCraryville\tNY\tColumbia County\tH1\n12062\t36021\tEast nassau\tNY\tColumbia County\tH1\n12546\t36021\tMillerton\tNY\tColumbia County\tH1\n12050\t36021\tColumbiaville\tNY\tColumbia County\tH1\n12173\t36021\tStuyvesant\tNY\tColumbia County\tH1\n12526\t36021\tGermantown\tNY\tColumbia County\tH1\n12156\t36021\tSchodack landing\tNY\tColumbia County\tH1\n12523\t36021\tElizaville\tNY\tColumbia County\tH1\n12530\t36021\tHollowville\tNY\tColumbia County\tH1\n12565\t36021\tPhilmont\tNY\tColumbia County\tH1\n12544\t36021\tMellenville\tNY\tColumbia County\tH1\n12132\t36021\tNorth chatham\tNY\tColumbia County\tH1\n12516\t36021\tCopake\tNY\tColumbia County\tH1\n12106\t36021\tKinderhook\tNY\tColumbia County\tH1\n12136\t36021\tOld chatham\tNY\tColumbia County\tH1\n12125\t36021\tNew lebanon\tNY\tColumbia County\tH1\n12567\t36021\tPine plains\tNY\tColumbia County\tH1\n12024\t36021\tBrainard\tNY\tColumbia County\tH1\n12017\t36021\tAusterlitz\tNY\tColumbia County\tH1\n12165\t36021\tSpencertown\tNY\tColumbia County\tH1\n12541\t36021\tLivingston\tNY\tColumbia County\tH1\n13053\t36023\tDryden\tNY\tCortland County\tH1\n13835\t36023\tRichford\tNY\tCortland County\tH1\n13803\t36023\tMarathon\tNY\tCortland County\tH1\n13841\t36023\tSmithville flats\tNY\tCortland County\tH1\n13141\t36023\tPreble\tNY\tCortland County\tH1\n13738\t36023\tBlodgett mills\tNY\tCortland County\tH1\n13101\t36023\tMc graw\tNY\tCortland County\tH1\n13040\t36023\tCincinnatus\tNY\tCortland County\tH1\n13045\t36023\tCortland\tNY\tCortland County\tH1\n13077\t36023\tHomer\tNY\tCortland County\tH1\n13073\t36023\tGroton\tNY\tCortland County\tH1\n13784\t36023\tHarford\tNY\tCortland County\tH1\n13052\t36023\tDe ruyter\tNY\tCortland County\tH1\n13862\t36023\tWhitney point\tNY\tCortland County\tH1\n13158\t36023\tTruxton\tNY\tCortland County\tH1\n13159\t36023\tTully\tNY\tCortland County\tH1\n13863\t36023\tWillet\tNY\tCortland County\tH1\n13087\t36023\tLittle york\tNY\tCortland County\tH1\n12455\t36025\tMargaretville\tNY\tDelaware County\tH1\n13731\t36025\tAndes\tNY\tDelaware County\tH1\n12434\t36025\tGrand gorge\tNY\tDelaware County\tH1\n12155\t36025\tSchenevus\tNY\tDelaware County\tH1\n13756\t36025\tEast branch\tNY\tDelaware County\tH1\n12406\t36025\tArkville\tNY\tDelaware County\tH1\n12459\t36025\tNew kingston\tNY\tDelaware County\tH1\n12758\t36025\tLivingston manor\tNY\tDelaware County\tH1\n12167\t36025\tStamford\tNY\tDelaware County\tH1\n13740\t36025\tBovina center\tNY\tDelaware County\tH1\n13846\t36025\tTreadwell\tNY\tDelaware County\tH1\n12093\t36025\tJefferson\tNY\tDelaware County\tH1\n13753\t36025\tDelhi\tNY\tDelaware County\tH1\n13849\t36025\tUnadilla\tNY\tDelaware County\tH1\n13786\t36025\tHarpersfield\tNY\tDelaware County\tH1\n13842\t36025\tSouth kortright\tNY\tDelaware County\tH1\n12776\t36025\tRoscoe\tNY\tDelaware County\tH1\n13754\t36025\tDeposit\tNY\tDelaware County\tH1\n13788\t36025\tHobart\tNY\tDelaware County\tH1\n13806\t36025\tMeridale\tNY\tDelaware County\tH1\n13755\t36025\tDownsville\tNY\tDelaware County\tH1\n13733\t36025\tBainbridge\tNY\tDelaware County\tH1\n13739\t36025\tBloomville\tNY\tDelaware County\tH1\n13839\t36025\tSidney center\tNY\tDelaware County\tH1\n13825\t36025\tOtego\tNY\tDelaware County\tH1\n13751\t36025\tDavenport center\tNY\tDelaware County\tH1\n12438\t36025\tHalcottsville\tNY\tDelaware County\tH1\n12474\t36025\tRoxbury\tNY\tDelaware County\tH1\n13782\t36025\tHamden\tNY\tDelaware County\tH1\n13838\t36025\tSidney\tNY\tDelaware County\tH1\n13856\t36025\tWalton\tNY\tDelaware County\tH1\n12465\t36025\tPine hill\tNY\tDelaware County\tH1\n13774\t36025\tFishs eddy\tNY\tDelaware County\tH1\n13757\t36025\tEast meredith\tNY\tDelaware County\tH1\n13847\t36025\tTrout creek\tNY\tDelaware County\tH1\n13783\t36025\tHancock\tNY\tDelaware County\tH1\n12421\t36025\tDenver\tNY\tDelaware County\tH1\n13752\t36025\tDelancey\tNY\tDelaware County\tH1\n13804\t36025\tMasonville\tNY\tDelaware County\tH1\n13750\t36025\tDavenport\tNY\tDelaware County\tH1\n13860\t36025\tWest 
